vi "p11.vi"() -> ()   [LabVIEW 2015]
uses:
  <vilib>/Analysis/Matrix/Datatypes/RealMatrix.ctl
  <vilib>/Analysis/Matrix/Numeric/Conversions/Matrix To Array - RM.vi
  <vilib>/Analysis/Matrix/NI_Matrix.lvlib
panel:
  out "SET : Submatrix":T1
  out "SET : Matrix Element":T1
  out "SET : Diagonal Matrix":T1
  out "submatrix":T1
  out "element":dbl
  out "Matrix Diagonal":T1
  out "transposed matrix":T1
  out "resized matrix":T1
  out "appended array 2":T1
  out "Matrix - Column":i32
  out "Matrix - Row":i32
  out "Real 2D Array":dbl[][](array[numeric])
  out "array":dbl[](array[numeric])
  in  "Cluster":T2
  out "Array to Cluster":T3
  out "interleaved array":dbl[](array[numeric])
  out "Value from Array":dbl
  out "Index w.r.t to Fractional Index":dbl
  out "decimated array 2":dbl[](array[numeric])
  out "decimated array 1":dbl[](array[numeric])
  out "array (last n elements first)":dbl[](array[numeric])
  out "reversed array":dbl[](array[numeric])
  out "transposed array":dbl[][](array[numeric])
  out "second subarray":dbl[](array[numeric])
  out "first subarray":dbl[](array[numeric])
  out "search index":i32
  out "Sorted Array":dbl[](array[numeric])
  out "Reshaped  Array":dbl[](array[numeric])
  out "min index(es)":i32
  out "min value":dbl
  out "max index(es)":i32
  out "max value":dbl
  out "subarray":dbl[](array[numeric])
  out "appended array":dbl[](array[numeric])
  out "initialized array":dbl[](array[numeric])
  out "output array":dbl[][](array[numeric])
  out "deleted portion":dbl[](array[numeric])
  out "array w/ subset deleted":dbl[][](array[numeric])
  out "Insert into 2D array":dbl[][](array[numeric])
  out "size of 2D array":i32[](array[numeric])
  out "Index":dbl
  out "Replaced Array":dbl[](array[numeric])
  out "deleted portion":dbl[](array[numeric])
  out "After deletion":dbl[](array[numeric])
  out "Insert into Array":dbl[](array[numeric])
  out "Index":dbl
  out "size(s)":i32
  # "EXAMPLE : ONE - DIMENSIONAL ARRAY"
  # "EXAMPLE : TWO - DIMENSIONAL ARRAY"
  # "SIZE OF AN ARRAY"
  # "DELETE FROM ARRAY"
  # "SIZE OF AN ARRAY"
  # "DELETE FROM ARRAY"
  # "INDEX OF AN ARRAY"
  # "INDEX OF AN ARRAY"
  # "INSERT INTO AN ARRAY"
  # "REPLACE AN ARRAY"
  # "REPLACE AN ARRAY"
  # "INSERT INTO AN ARRAY"
  # "TRANSPOSE OF AN ARRAY"
  # "MATRIX ---> 2D ARRAY"
  # "INITIALIZE ARRAY"
  # "SUBSET OF AN ARRAY"
  # "MAX & MIN OF ARRAY"
  # "EXAMPLE : MATRIX"
  # "BULD AN ARRAY"
  # "RESHAPE AN ARRAY"
  # "SORT AN ARRAY"
  # "SIZE OF MATRIX"
  # "DIAGONAL MATRIX OF R & C"
  # "SET DIAGONAL MATRIX OF R & C"
  # "APPEND MATRIX"
  # "GET MATRIX ELEMENT"
  # "SEARCH AN ELEMENT \nIN AN ARRAY"
  # "SUBMATRIX OF R & C"
  # "SUBSET AN ARRAY"
  # "REVERSE AN ARRAY"
  # "RESIZE MATRIX"
  # "SET MATRIX ELEMENT"
  # "ROTATE \"n\"  AN ARRAY"
  # "INTERPOLATE 1D ARRAY"
  # "TRANSPOSE A MATRIX"
  # "INTERPOLATE 1D ARRAY"
  # "SET SUBMATRIX"
  # "DECIMINATE AN ARRAY"
  # "INTERLEAVED ARRAY"
  # "CLUSTER TO ARRAY"
  # "ARRAY TO CLUSTER"
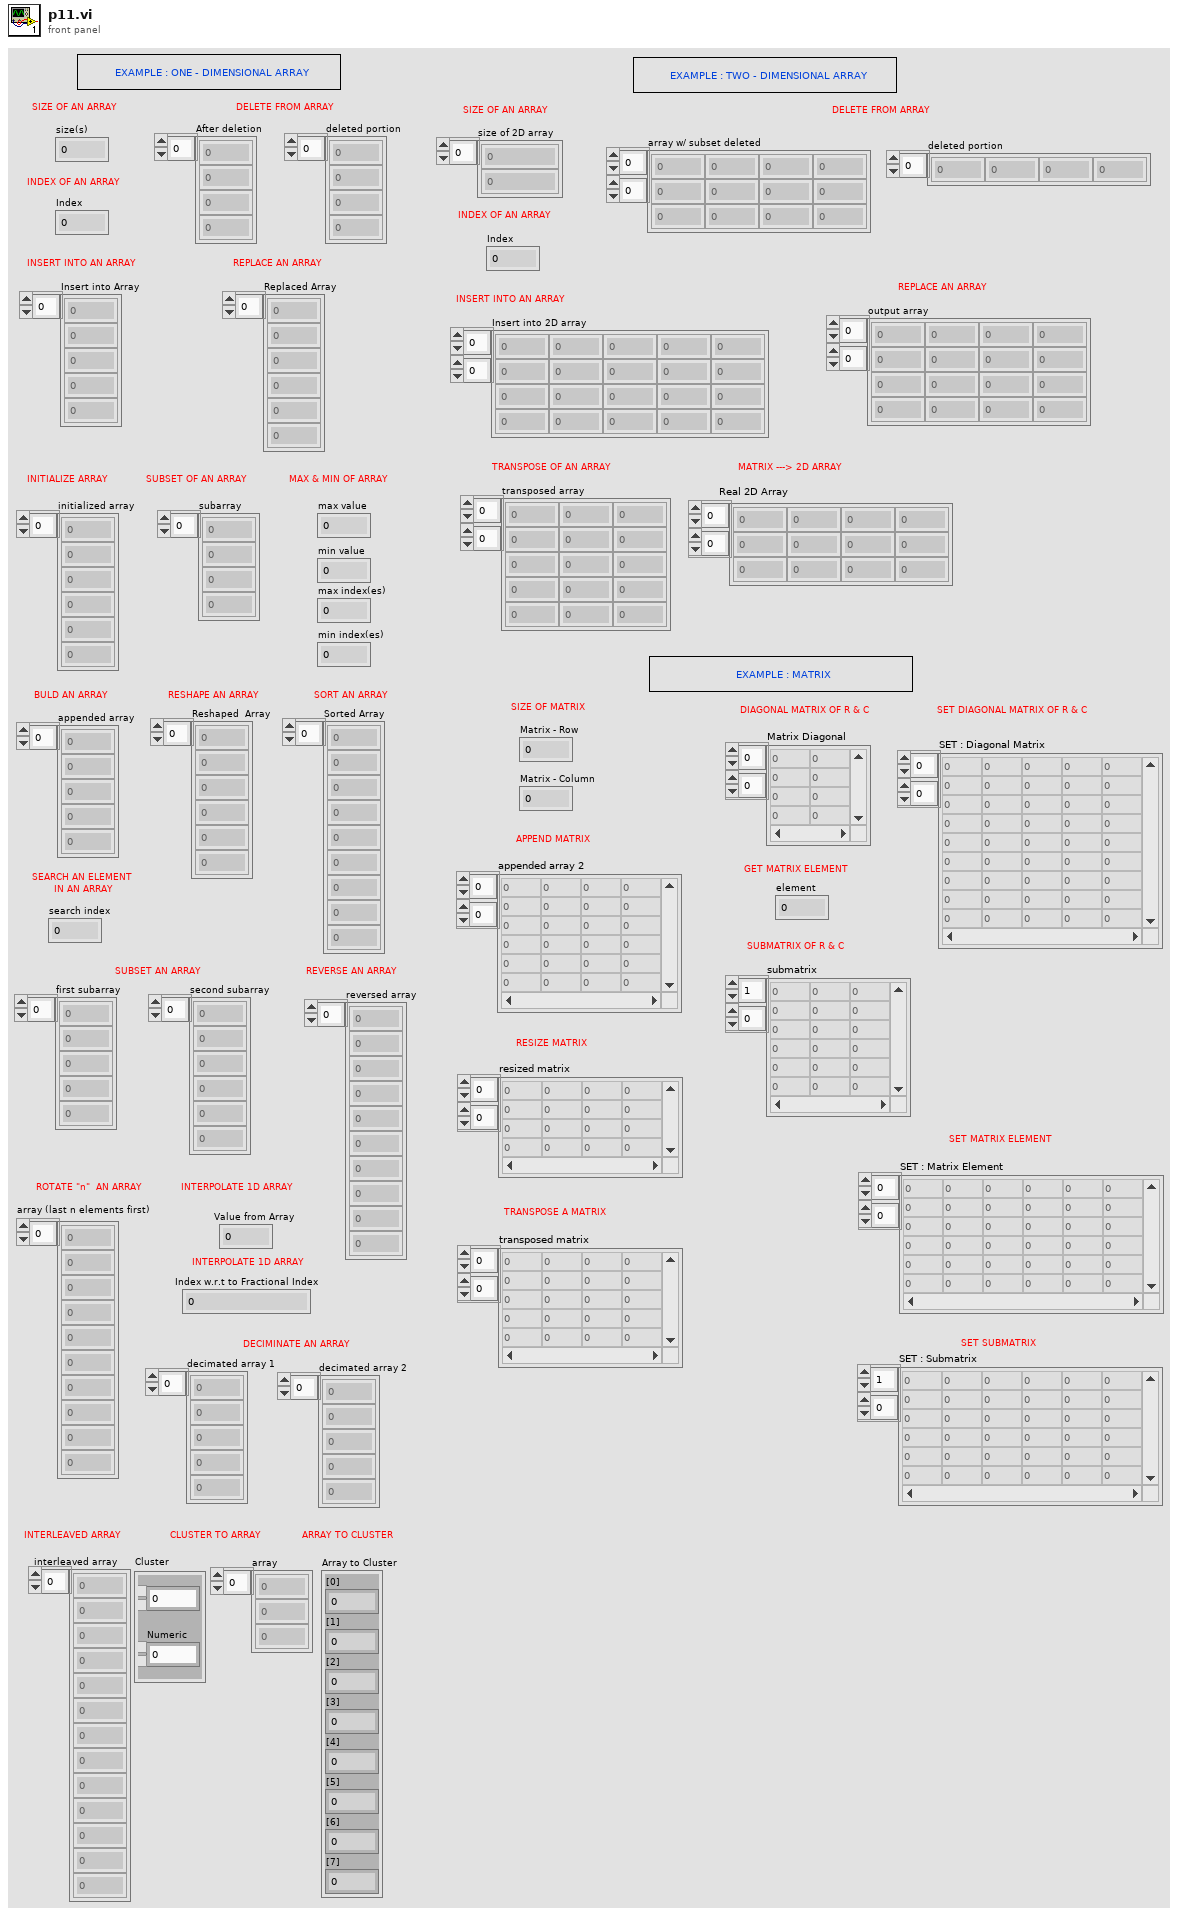
[diagram p1: front panel]
types:
  T1 = typedef "NI_Matrix.lvlib/RealMatrix.ctl" = dbl[][]
  T2 = cluster{"Real Matrix Element":dbl, "Numeric":dbl}
  T3 = cluster{"[0]":i32, "[1]":i32, "[2]":i32, "[3]":i32, "[4]":i32, "[5]":i32, "[6]":i32, "[7]":i32}
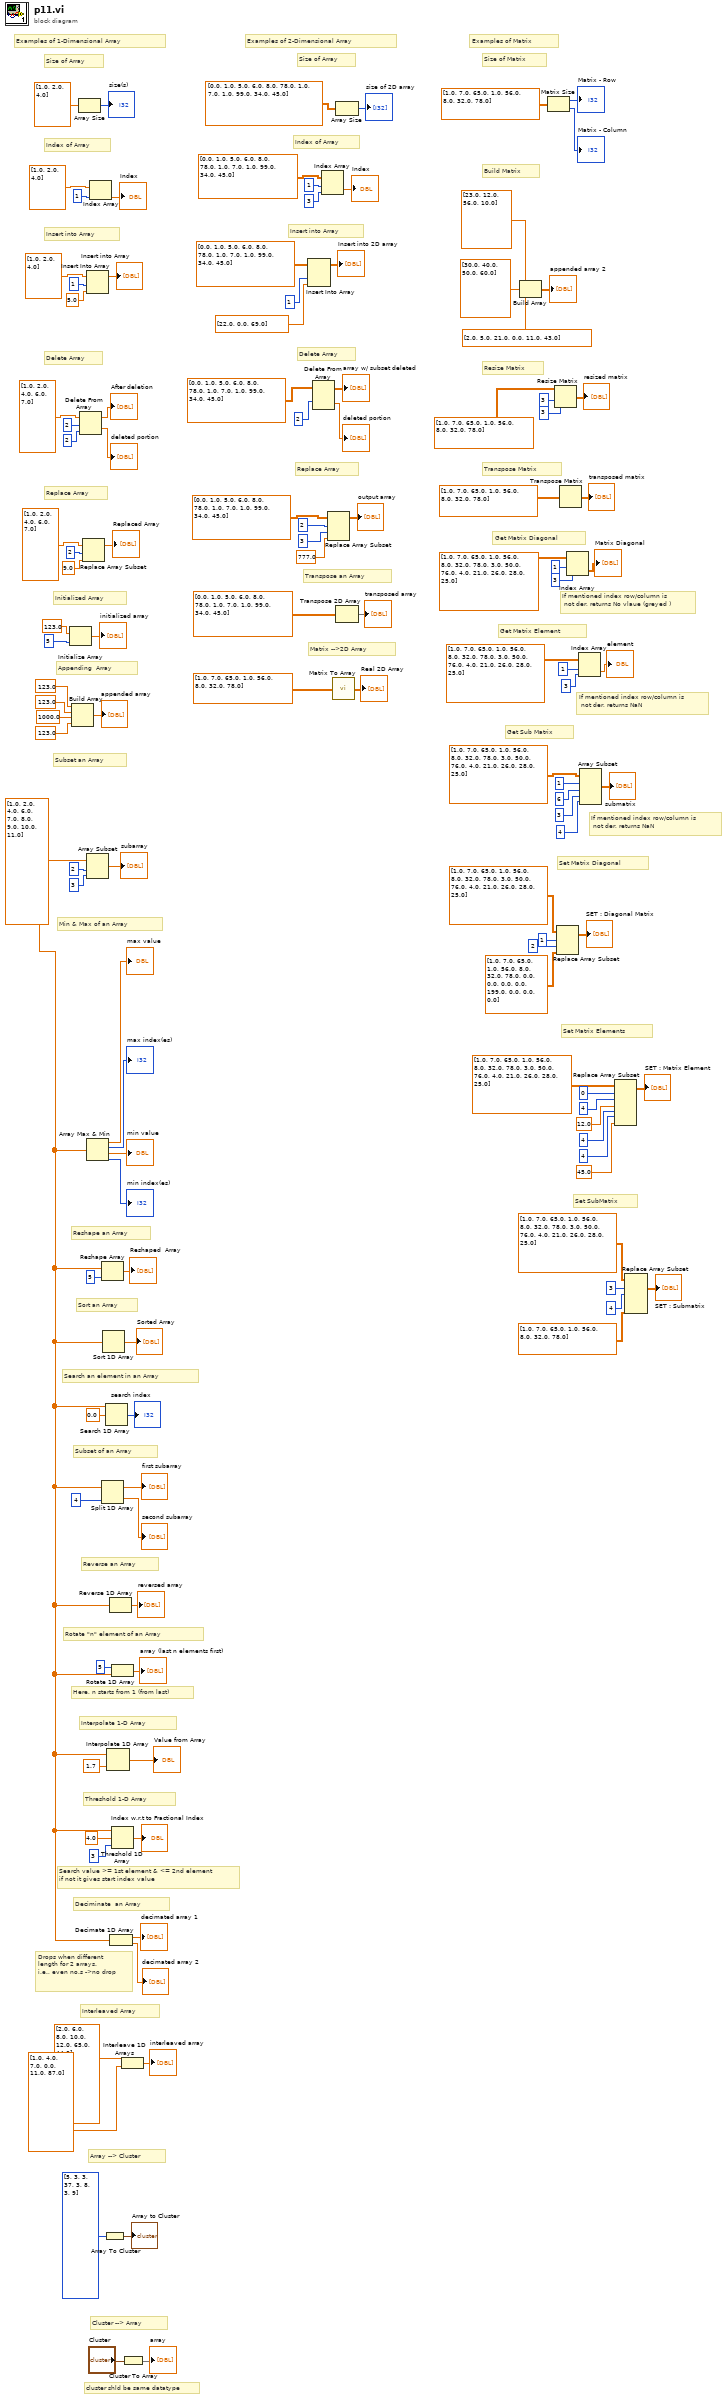
[diagram p0: block diagram]
diagram:
  w57 = dbl[] [1.0, 2.0, 4.0, 6.0, 7.0, 8.0, 9.0, 10.0, 11.0] ("element")
  # "Set SubMatrix"
  # "Set Matrix Elements"
  # "Set Matrix Diagonal"
  # "Get Sub Matrix"
  # "Get Matrix Element"
  # "Get Matrix Diagonal"
  # "If mentioned index row/column is\n not der, returns No vlaue (greyed )"
  # "If mentioned index row/column is\n not der, returns NaN"
  # "If mentioned index row/column is\n not der, returns NaN"
  # "Transpose Matrix"
  # "Resize Matrix"
  # "Build Matrix"
  # "Size of Matrix"
  # "Examples of Matrix"
  # "Matrix -->2D Array"
  # "Transpose an Array"
  # "cluster shld be same datatype"
  # "Interleaved Array"
  # "Array --> Cluster"
  # "Cluster --> Array"
  # "Search value >= 1st element & <= 2nd element\nif not it gives start index value"
  # "Deciminate  an Array"
  # "Threshold 1-D Array"
  # "Interpolate 1-D Array"
  # "Drops when different length for 2 arrays.\ni.e., even no.s ->no drop"
  # "Rotate \"n\" element of an Array"
  # "Reverse an Array"
  # "Subset of an Array"
  # "Search an element in an Array"
  # "Sort an Array"
  # "Reshape an Array"
  # "Here, n starts from 1 (from last)"
  # "Initialized Array"
  # "Min & Max of an Array"
  # "Subset an Array"
  # "Appending  Array"
  # "Replace Array"
  # "Delete Array"
  # "Insert into Array"
  # "Index of Array"
  # "Size of Array"
  # "Examples of 2-Dimensional Array"
  # "Examples of 1-Dimensional Array"
  # "Replace Array"
  # "Delete Array"
  # "Insert into Array"
  # "Index of Array"
  # "Size of Array"
  n1 = Initialize Array(123.0 ("element"), 5 ("dimension size")) -> (→"initialized array":dbl[])
  n2 = Build Array(123.0 ("element"), 123.0 ("element"), 1000.0 ("element"), 123.0 ("element")) -> (→"appended array":dbl[])
  n3 = Array Size(array=dbl[] [1.0, 2.0, 4.0] ("element")) -> (size(s)=→"size(s)":i32)
  n4 = Delete From Array(array=dbl[] [1.0, 2.0, 4.0, 6.0, 7.0] ("element"), length=2, index=2) -> (deleted portion=→"deleted portion":dbl[], array with subset deleted=→"After deletion":dbl[])
  n5 = Replace Array Subset(array=dbl[] [1.0, 2.0, 4.0, 6.0, 7.0] ("element"), new element=9.0 ("new element/subarray"), index=2) -> (→"Replaced Array":dbl[])
  n6 = Insert Into Array(array=dbl[] [1.0, 2.0, 4.0] ("element"), index=1, new element=5.0 ("new element/subarray")) -> (→"Insert into Array":dbl[])
  n7 = Array Subset(array=w57, index=2, length=3 ("index")) -> (→"subarray":dbl[])
  n8 = Array Max & Min(array=w57) -> (max value=→"max value":dbl, max index (indices)=→"max index(es)":i32, min value=→"min value":dbl, min index (indices)=→"min index(es)":i32)
  n9 = Index Array(array=dbl[] [1.0, 2.0, 4.0] ("element"), index=1) -> (element=→"Index":dbl)
  n10 = Reshape Array(w57, 5 ("dimension size")) -> (→"Reshaped  Array":dbl[])
  n11 = Split 1D Array(array=w57, index=4) -> (first subarray=→"first subarray":dbl[], second subarray=→"second subarray":dbl[])
  n12 = Sort 1D Array(array=w57) -> (sorted array=→"Sorted Array":dbl[])
  n13 = Array To Cluster(array=i32[] [5, 3, 3, 37, 3, 8, 3, 9]) -> (cluster=→"Array to Cluster":T3)
  n14 = Search 1D Array(1D array=w57, element=0.0) -> (index of element=→"search index":i32)  [unwired: 1 in]
  n15 = Interpolate 1D Array(1:1.7 ("fractional index or x"), 2:w57) -> (0:→"Value from Array":dbl)
  n16 = Reverse 1D Array(array=w57) -> (reversed array=→"reversed array":dbl[])
  n17 = Decimate 1D Array(w57) -> (→"decimated array 1":dbl[], →"decimated array 2":dbl[])
  n18 = Rotate 1D Array(1:w57, 2:5 ("n")) -> (0:→"array (last n elements first)":dbl[])
  n19 = Threshold 1D Array(1:3 ("start index (0)"), 2:4.0 ("threshold y"), 3:w57) -> (0:→"Index w.r.t to Fractional Index":dbl)
  n20 = Interleave 1D Arrays(dbl[] [2.0, 6.0, 8.0, 10.0, 12.0, 65.0, 44.0] ("decimated array 4"), dbl[] [1.0, 4.0, 7.0, 0.0, 11.0, 87.0] ("decimated array 3")) -> (→"interleaved array":dbl[])
  n21 = Cluster To Array(cluster="Cluster") -> (array=→"array":dbl[])
  n22 = Insert Into Array(array=dbl[][] [[0.0, 1.0, 5.0, 6.0], [8.0, 78.0, 1.0, 7.0], [1.0, 99.0, 34.0, 45.0]], index (col)=1 ("disabled index (col)"), new element=dbl[] [22.0, 0.0, 69.0] ("Real Matrix Element")) -> (→"Insert into 2D array":dbl[][])  [unwired: 1 in]
  n23 = Delete From Array(array=dbl[][] [[0.0, 1.0, 5.0, 6.0], [8.0, 78.0, 1.0, 7.0], [1.0, 99.0, 34.0, 45.0]], index (row)=2 ("length")) -> (deleted portion=→"deleted portion":dbl[], array with subset deleted=→"array w/ subset deleted":dbl[][])  [unwired: 2 in]
  n24 = Index Array(array=dbl[][] [[0.0, 1.0, 5.0, 6.0], [8.0, 78.0, 1.0, 7.0], [1.0, 99.0, 34.0, 45.0]], index (row)=1 ("index"), index (col)=3 ("disabled index (col)")) -> (element=→"Index":dbl)
  n25 = Replace Array Subset(array=dbl[][] [[0.0, 1.0, 5.0, 6.0], [8.0, 78.0, 1.0, 7.0], [1.0, 99.0, 34.0, 45.0]], new element=777.0 ("new element/subarray"), index (row)=2 ("index"), index (col)=3 ("disabled index (col)")) -> (→"output array":dbl[][])
  n26 = call-poly <vilib>:"Matrix To Array.vi"("Real Matrix"=T1 [[1.0, 7.0, 65.0, 1.0], [56.0, 8.0, 32.0, 78.0]]) -> ("Real 2D Array"=→"Real 2D Array":dbl[][])
  n27 = Array Size(array=dbl[][] [[0.0, 1.0, 5.0, 6.0], [8.0, 78.0, 1.0, 7.0], [1.0, 99.0, 34.0, 45.0]]) -> (size(s)=→"size of 2D array":i32[])
  n28 = Transpose 2D Array(2D array=dbl[][] [[0.0, 1.0, 5.0, 6.0], [8.0, 78.0, 1.0, 7.0], [1.0, 99.0, 34.0, 45.0]]) -> (transposed array=→"transposed array":dbl[][])
  n29 = Build Array(dbl[] [23.0, 12.0, 56.0, 10.0] ("element"), dbl[] [30.0, 40.0, 50.0, 60.0] ("element"), dbl[] [2.0, 5.0, 21.0, 0.0, 11.0, 43.0] ("element")) -> (→"appended array 2":T1)
  n30 = Matrix Size(0:T1 [[1.0, 7.0, 65.0, 1.0], [56.0, 8.0, 32.0, 78.0]] ("Real Matrix")) -> (1:→"Matrix - Row":i32, 2:→"Matrix - Column":i32)
  n31 = Resize Matrix(1:3 ("number of columns"), 2:3 ("number of rows"), 4:T1 [[1.0, 7.0, 65.0, 1.0], [56.0, 8.0, 32.0, 78.0]] ("Real Matrix")) -> (0:→"resized matrix":T1)
  n32 = Replace Array Subset(array=T1 [[1.0, 7.0, 65.0, 1.0], [56.0, 8.0, 32.0, 78.0], [3.0, 50.0, 76.0, 4.0], [21.0, 26.0, 28.0, 25.0]] ("Real Matrix"), new element=T1 [[1.0, 7.0, 65.0, 1.0], [56.0, 8.0, 32.0, 78.0], [0.0, 0.0, 0.0, 0.0], [199.0, 0.0, 0.0, 0.0]] ("Real Matrix"), index (row)=1 ("index (col)"), index (col)=2 ("disabled index (col)")) -> (→"SET : Diagonal Matrix":T1)
  n33 = Transpose Matrix(1:T1 [[1.0, 7.0, 65.0, 1.0], [56.0, 8.0, 32.0, 78.0]] ("Real Matrix")) -> (0:→"transposed matrix":T1)
  n34 = Index Array(array=T1 [[1.0, 7.0, 65.0, 1.0], [56.0, 8.0, 32.0, 78.0], [3.0, 50.0, 76.0, 4.0], [21.0, 26.0, 28.0, 25.0]] ("Real Matrix"), index (row)=1, index (col)=3) -> (element=→"Matrix Diagonal":T1)
  n35 = Index Array(array=T1 [[1.0, 7.0, 65.0, 1.0], [56.0, 8.0, 32.0, 78.0], [3.0, 50.0, 76.0, 4.0], [21.0, 26.0, 28.0, 25.0]] ("Real Matrix"), index (row)=1 ("index (col)"), index (col)=3) -> (element=→"element":dbl)
  n36 = Array Subset(array=T1 [[1.0, 7.0, 65.0, 1.0], [56.0, 8.0, 32.0, 78.0], [3.0, 50.0, 76.0, 4.0], [21.0, 26.0, 28.0, 25.0]] ("Real Matrix"), index (row)=1 ("index (col)"), length (row)=6 ("index (col)"), index (col)=3, length (col)=4 ("index (col)")) -> (→"submatrix":T1)
  n37 = Replace Array Subset(array=T1 [[1.0, 7.0, 65.0, 1.0], [56.0, 8.0, 32.0, 78.0], [3.0, 50.0, 76.0, 4.0], [21.0, 26.0, 28.0, 25.0]] ("Real Matrix"), new element #1=12.0 ("index (col)"), index (row) #1=0 ("index (col)"), index (col) #1=4 ("index (col)"), new element #2=45.0 ("index (col)"), index (row) #2=4 ("index (col)"), index (col) #2=4 ("index (col)")) -> (→"SET : Matrix Element":T1)
  n38 = Replace Array Subset(array=T1 [[1.0, 7.0, 65.0, 1.0], [56.0, 8.0, 32.0, 78.0], [3.0, 50.0, 76.0, 4.0], [21.0, 26.0, 28.0, 25.0]] ("Real Matrix"), new element=T1 [[1.0, 7.0, 65.0, 1.0], [56.0, 8.0, 32.0, 78.0]] ("Real Matrix"), index (dim 0)=3 ("index (col)"), index (dim 1)=4 ("index (col)")) -> (→"SET : Submatrix":T1)  [unwired: 2 in]
